vi "Start Async.vi"(8 "error in (no error)":errorcluster, 11 "gRPC service in":refnum<class "Template.lvclass">) -> (0 "error out":errorcluster, 3 "gRPC service out":refnum<class "Template.lvclass">)   [LabVIEW 2021, in "Template_server.lvlib" / "Template.lvclass"]
uses:
  Template.lvclass
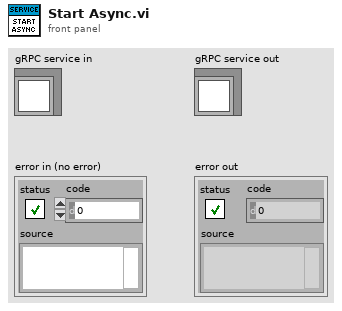
[diagram p1: front panel]
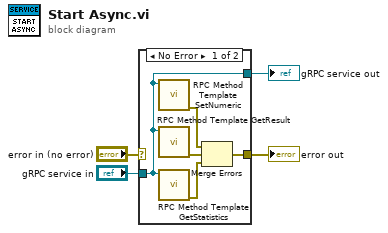
[diagram p0: block diagram]
diagram:
  n1 = case shown="No Error" "error in (no error)" {
    selector: "error in (no error)" -> [_ w11]
    tunnel: [w9 w11] -> w3
    tunnel: [w8 w10] -> w1
    tunnel: "gRPC service in" -> [w8 w10]
    frame No Error {
      n2 = call "RPC Method Template SetNumeric.vi"("gRPC service in"=w8) -> ("error out"=w7:errorcluster)  [unwired: 9 in, 1 out]
      n3 = call "RPC Method Template GetResult.vi"("gRPC service in"=w8) -> ("error out"=w6:errorcluster)  [unwired: 9 in, 1 out]
      n4 = call "RPC Method Template GetStatistics.vi"("gRPC service in"=w8) -> ("error out"=w5:errorcluster)  [unwired: 9 in, 1 out]
      n5 = Merge Errors(w7, w6, w5) -> (w9:errorcluster)
    }
    frame Error {
    }
  }
  "error out" <- w3
  "gRPC service out" <- w1
